vi "Increment Skipped Count.vi"(8 "error in (no error)":errorcluster, 11 "Result Table.lvclass":refnum<class "Result Table.lvclass">) -> (0 "error out":errorcluster, 3 "Result Table":refnum<class "Result Table.lvclass">)   [LabVIEW 2020, in "Result Table.lvclass"]
uses:
  Result Table.lvclass
  TypeDefs/Table Columns.ctl
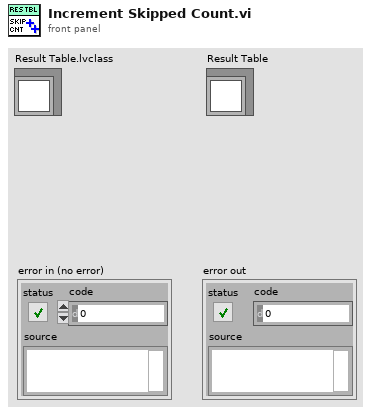
[diagram p1: front panel]
types:
  T1 = typedef "Result Table.lvclass/Table Columns.ctl" = u16
  T2 = typedef "Result Table.lvclass/Results.ctl" = cluster{"Method Count":u32, "Executed Methods":u32, "Passed Methods":u32, "Failed Methods":u32, "Method Errors":u32, "Skipped Method":u32}
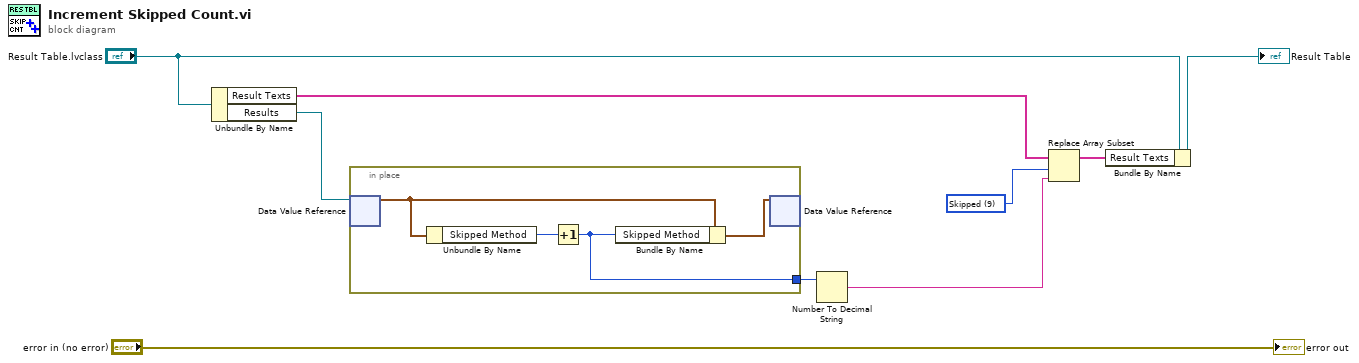
[diagram p0: block diagram]
diagram:
  w3 = T1 9 items=["Last run:"=1, "Passed:"=3, "Failed:"=5, "Errors:"=7, "Skipped"=9] ("Table Columns")
  n1 = Unbundle By Name("Result Table.lvclass") -> ("Result Texts"=w4:string[], "Results"=w8:refnum<data-value>)
  n2 = in-place {
    in-place-border: [w10] -> w7
    n3 = in-place-dvr #1(w8) -> (w12:T2)  [unwired: 1 out]
    n4 = Unbundle By Name(w12) -> ("Skipped Method"=w11:u32)
    n5 = Increment(x=w11) -> (x+1=w10:u32)
    n6 = Bundle By Name(cluster=w12, "Skipped Method"=w10) -> (w13:T2)
    n7 = in-place-dvr #1(w13) -> ()  [unwired: 2 out]
  }
  n8 = Number To Decimal String(number=w7) -> (decimal integer string=w6:string)  [unwired: 1 in]
  n9 = Replace Array Subset(array=w4, new element=w6, index=w3) -> (w1:string[])
  n10 = Bundle By Name(cluster="Result Table.lvclass", "Result Texts"=w1) -> (→"Result Table":refnum<class "Result Table.lvclass">)
  "error out" <- "error in (no error)"
